vi "String.Compare to Patterns.vi"(5 "Case Insensitive":bool, 7 "Comparison":enum16{"Contains", "Starts With", "Ends With"}(ring), 10 "Patterns":string[](array[string]), 11 "String In":string) -> (3 "Match":bool)   [LabVIEW 2019]
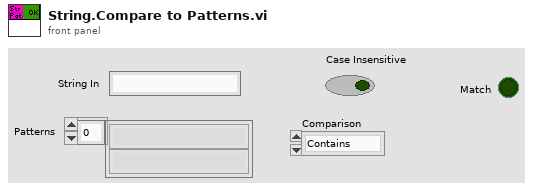
[diagram p1: front panel]
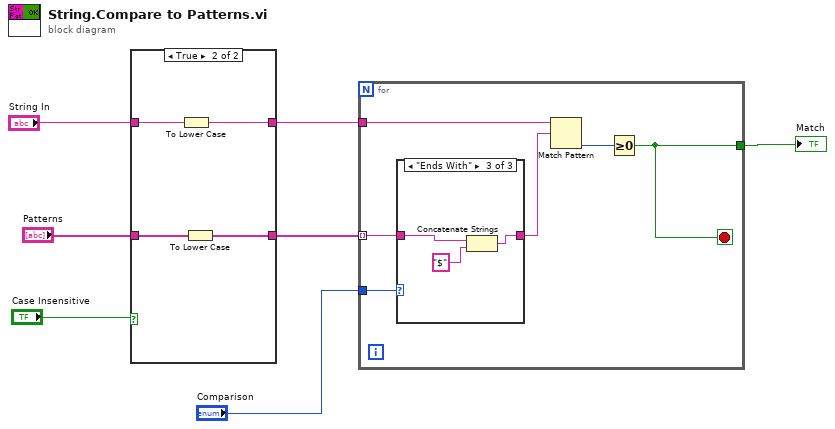
[diagram p0: block diagram]
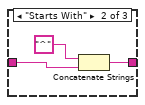
[diagram p4: hidden frame]
diagram:
  n1 = case shown="True" "Case Insensitive" {
    tunnel: "Patterns" -> [w8 w13]
    tunnel: "String In" -> [w9 w12]
    tunnel: [w9 w11] -> w4
    tunnel: [w8 w10] -> w3
    frame False {
    }
    frame True {
      n2 = To Lower Case(string=w12) -> (all lower case string=w11:string)
      n3 = To Lower Case(string=w13) -> (all lower case string=w10:string[])
    }
  }
  n4 = for {
    tunnel: w4 -> [w19]
    tunnel: w3 -> [w15] mode=indexing
    tunnel: [w17] -> w2
    tunnel: "Comparison" -> [w16]
    stop <- w17 stop-if-true
    n5 = case shown="\"Ends With\"" w16 {
      tunnel: w15 -> [w20 w22 w25]
      tunnel: [w20 w23 w26] -> w14
      frame "Contains", Default {
      }
      frame "Starts With" {
        n6 = Concatenate Strings("^" ("string"), w22) -> (w23:string)
      }
      frame "Ends With" {
        n7 = Concatenate Strings(w25, "$" ("string")) -> (w26:string)
      }
    }
    n8 = Match Pattern(string=w19, regular expression=w14) -> (offset past match=w18:i32)  [unwired: 1 in, 3 out]
    n9 = Greater Or Equal To 0?(x=w18) -> (x >= 0?=w17:bool)
  }
  "Match" <- w2
